vi "Step Add -DCW W Parameters.vi"(0 "VISA resource name":refnum<visa-resource-name>, 2 "Internal Scanner Exists?":bool, 3 "Scanner Settings":T2={"Scan1"=1, "Scan2"=1, "Scan3"=1, "Scan4"=1, "Scan5"=1, "Scan6"=1, "Scan7"=1, "Scan8"=1, "Scan9"=1, "Scan10"=1, "Scan11"=1, "Scan12"=1, "Scan13"=1, "Scan14"=1, "Scan15"=1, "Scan16"=1} {"Scan16" scale=0.0..2.0; "Scan15" scale=0.0..2.0; "Scan14" scale=0.0..2.0; "Scan13" scale=0.0..2.0; "Scan12" scale=0.0..2.0; "Scan11" scale=0.0..2.0; "Scan10" scale=0.0..2.0; "Scan9" scale=0.0..2.0; "Scan8" scale=0.0..2.0; "Scan7" scale=0.0..2.0; "Scan6" scale=0.0..2.0; "Scan5" scale=0.0..2.0; "Scan4" scale=0.0..2.0; "Scan3" min=0 max=2 scale=0.0..2.0; "Scan2" min=0 max=2 scale=0.0..2.0; "Scan1" min=0 max=2 scale=0.0..2.0}, 7 "Step Selection (1-200)":i32=1, 9 "Add Step":bool, 11 "error in (no error)":errorcluster) -> (4 "VISA resource name out":refnum<visa-resource-name>, 15 "error out":errorcluster)   [LabVIEW 2020, in "Associated Research 78XX Series.lvlib"]
doc: "Set the desired memory location to DCW mode with the specified parameters."
uses:
  <instrlib>/Associated Research 78XX Series/Associated Research 78XX Series.lvlib
  <instrlib>/Associated Research 78XX Series/Public/Configure/Steps/Low Level/Scanner Settings.ctl
  <instrlib>/Associated Research 78XX Series/Public/Configure/Steps/Low Level/-DCW Test Parameters.ctl
panel:
  in  "DCW Test Parameters (in)":T1={"Voltage (-1500)"=-1500, "High Limit(0.0 - -10,000 microamps) (-10)"=-10000.0, "Low Limit(0.0 - -10,000 microamps) (0)"=0.0, "Ramp Up Time (0.4 - 999.9 seconds) (0.4)"=0.4, "Dwell Time (0, 0.4 - 999.9 seconds) (1)"=1.0, "Ramp Down Time (0, 1.0 - 999.9 seconds) (0) "=0.0, "Charge LO (0.0 - 350uA)"=0.0, "Arc Sense (1 - 9) (5)"=5, "Arc Detect (F: Off)"=FALSE, "Continuity (F: Off)"=FALSE, "Auto Charge LO (F: Off)"=FALSE, "Low Range (F: Off)"=FALSE, "Offset (0.0 - 10,000uA)"=0.0, "Ramp-Hi (0.0 - 10,000uA)"=0.0, "Range (F: AUTO)"=enum."AUTO"} {"Ramp-Hi (0.0 - 10,000uA)" format="%.2f"; "Offset (0.0 - 10,000uA)" format="%.2f"; "Ramp Down Time (0, 1.0 - 999.9 seconds) (0)" format="%.1f"; "Charge LO (0.0 - 350uA)" format="%.2f"; "Dwell Time (0, 0.4 - 999.9 seconds) (1)" format="%.1f"; "Ramp Up Time (0.4 - 999.9 seconds) (0.4)" format="%.1f"; "Low Limit(0.0 - -10,000 microamps) (0)" format="%.1f"; "High Limit(0.0 - -10,000 microamps) (-10)" format="%.1f"}
  # "Add"
  # "Edit"
  # "On\nOff"
  # "On\nOff"
  # "On\nOff"
  # "Fixed\nAuto"
  # "On\nOff"
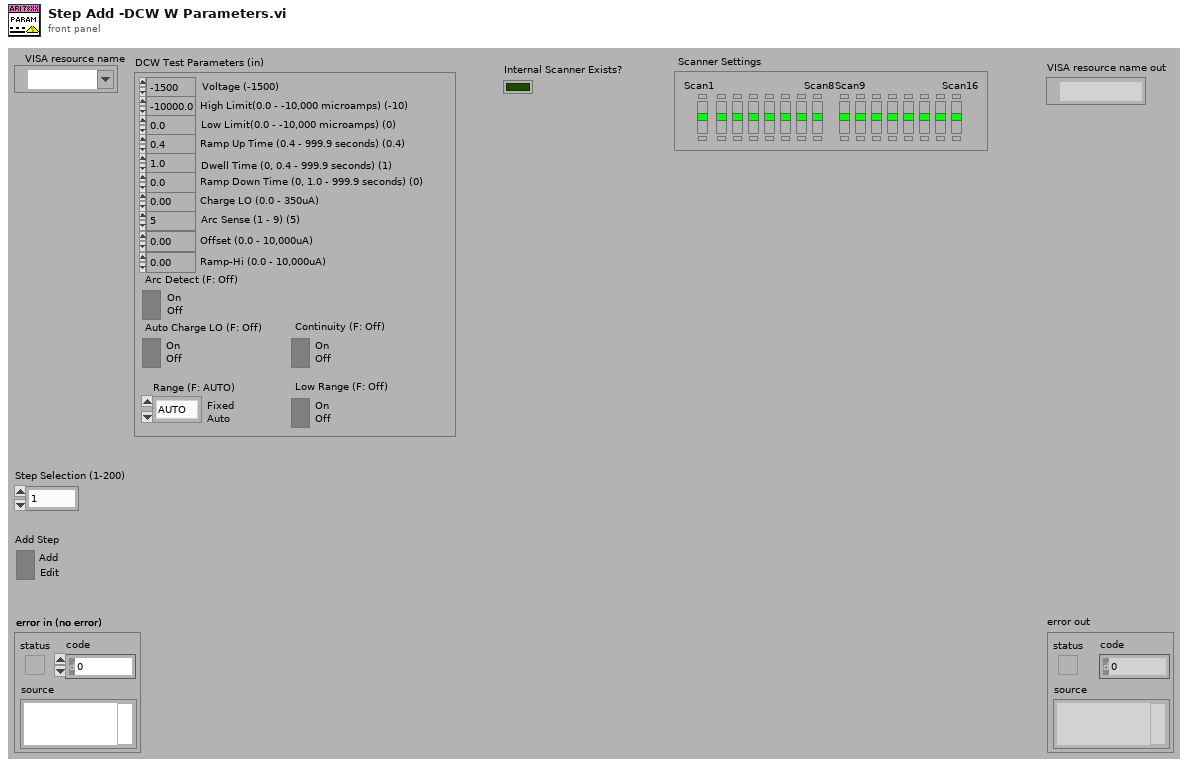
[diagram p1: front panel]
types:
  T1 = typedef "Associated Research 78XX Series.lvlib/-DCW Test Parameters.ctl" = cluster{"Voltage (-1500)":i32, "High Limit(0.0 - -10,000 microamps) (-10)":dbl, "Low Limit(0.0 - -10,000 microamps) (0)":dbl, "Ramp Up Time (0.4 - 999.9 seconds) (0.4)":dbl, "Dwell Time (0, 0.4 - 999.9 seconds) (1)":dbl, "Ramp Down Time (0, 1.0 - 999.9 seconds) (0) ":dbl, "Charge LO (0.0 - 350uA)":dbl, "Arc Sense (1 - 9) (5)":i32, "Arc Detect (F: Off)":bool, "Continuity (F: Off)":bool, "Auto Charge LO (F: Off)":bool, "Low Range (F: Off)":bool, "Offset (0.0 - 10,000uA)":dbl, "Ramp-Hi (0.0 - 10,000uA)":dbl, "Range (F: AUTO)":enum16{"AUTO", "FIXED"}}
  T2 = typedef "Associated Research 78XX Series.lvlib/Scanner Settings.ctl" = cluster{"Scan1":i32, "Scan2":i32, "Scan3":i32, "Scan4":i32, "Scan5":i32, "Scan6":i32, "Scan7":i32, "Scan8":i32, "Scan9":i32, "Scan10":i32, "Scan11":i32, "Scan12":i32, "Scan13":i32, "Scan14":i32, "Scan15":i32, "Scan16":i32}
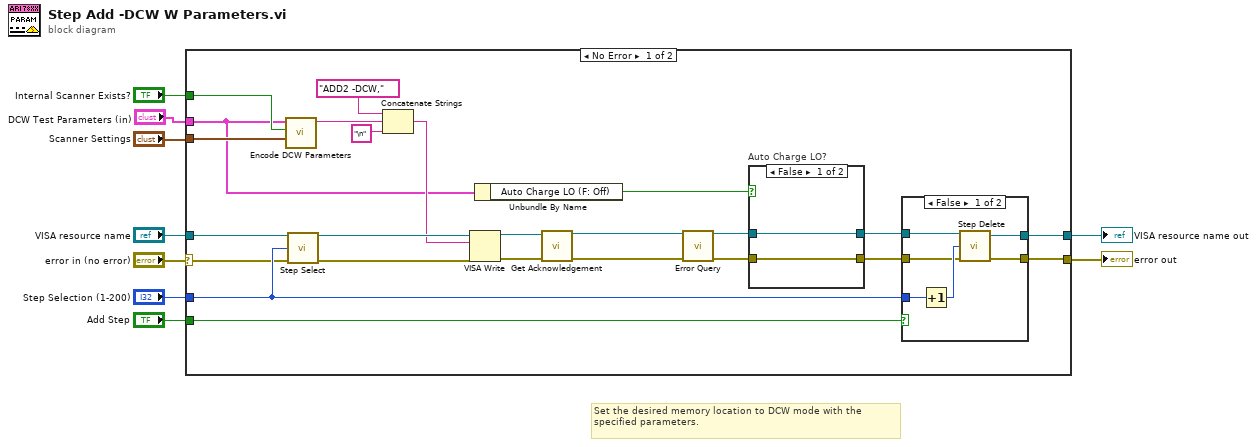
[diagram p0: block diagram]
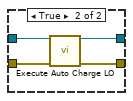
[diagram p2: hidden frame]
diagram:
  # "Set the desired memory location to DCW mode with the specified parameters."
  n1 = case shown="No Error" "error in (no error)" {
    selector: "error in (no error)" -> [w13 w49]
    tunnel: [w30 w49] -> w8
    tunnel: [w29 w48] -> w6
    tunnel: "VISA resource name" -> [w14 w48]
    tunnel: "Step Selection (1-200)" -> [w31 _]
    tunnel: "Add Step" -> [w28 _]
    tunnel: "DCW Test Parameters (in)" -> [w17 _]
    tunnel: "Internal Scanner Exists?" -> [w27 _]
    tunnel: "Scanner Settings" -> [w19 _]
    frame No Error {
      n2 = call <instrlib>:"Encode DCW Parameters.vi"("Scanner Settings"=w19, "Internal Scanner Exists?"=w27, "DCW Test Parameters out"=w17) -> ("Add Parameters"=w26:string)  [unwired: 6 in, 2 out]
      n3 = call <instrlib>:"Step Select.vi"("VISA resource name"=w14, "Step Number (1)"=w31, "error in (no error)"=w13) -> ("VISA resource name out"=w32:refnum<visa-resource-name>, "error out"=w33:errorcluster)  [unwired: 11 in]
      n4 = Concatenate Strings("ADD2 -DCW," ("string"), w26, "\n" ("string")) -> (w24:string)
      n5 = VISA Write(VISA resource name=w32, write buffer=w24, error in (no error)=w33) -> (VISA resource name out=w11:refnum<visa-resource-name>, error out=w10:errorcluster)  [unwired: 1 out]
      n6 = Unbundle By Name(w17) -> ("Auto Charge LO (F: Off)"=w18:bool)
      n7 = call <instrlib>:"Get Acknowledgement.vi"("VISA resource name"=w11, "error in (no error)"=w10) -> ("VISA resource name out"=w16:refnum<visa-resource-name>, "error out"=w15:errorcluster)  [unwired: 12 in]
      n8 = call <instrlib>:"Error Query.vi"("VISA resource name"=w16, "error in (no error)"=w15) -> ("VISA resource name out"=w23:refnum<visa-resource-name>, "error out"=w22:errorcluster)  [unwired: 10 in, 2 out]
      n9 = case "Auto Charge LO?" shown="False" w18 {
        tunnel: w23 -> [w35 w39]
        tunnel: w22 -> [w34 w38]
        tunnel: [w34 w36] -> w21
        tunnel: [w35 w37] -> w20
        frame False {
        }
        frame True {
          n10 = call <instrlib>:"Execute Auto Charge LO.vi"("VISA resource name"=w39, "error in (no error)"=w38) -> ("VISA resource name out"=w37:refnum<visa-resource-name>, "error out"=w36:errorcluster)  [unwired: 12 in]
        }
      }
      n11 = case shown="False" w28 {
        tunnel: w31 -> [w45 _]
        tunnel: w21 -> [w43 w46]
        tunnel: w20 -> [w42 w47]
        tunnel: [w41 w46] -> w30
        tunnel: [w40 w47] -> w29
        frame False {
          n12 = Increment(x=w45) -> (x+1=w44:i32)
          n13 = call <instrlib>:"Step Delete.vi"("VISA resource name"=w42, "Step Number (0 = Active Step)"=w44, "error in (no error)"=w43) -> ("VISA resource name out"=w40:refnum<visa-resource-name>, "error out"=w41:errorcluster)  [unwired: 11 in]
        }
        frame True {
        }
      }
    }
    frame Error {
    }
  }
  "error out" <- w8
  "VISA resource name out" <- w6
